vi "Test InfluxDB Client.vi"() -> ()   [LabVIEW 2015]
doc: "Test program for the InfluxDB client."
uses:
  Schema.ctl
  InfluxDB Client/InfluxDB Client.lvclass
  InfluxDB Client/Time precision.ctl
panel:
  out "Data out":T1[](array[typedef]) {"time" format="%<%I:%M:%S%3u %p\n%Y/%m/%d>T"}
  in  "Data in":T1[](array[typedef])=[{"time"=timestamp(3513058155.541 s since 1904-01-01), "string"="textA", "extended"=1.234, "double"=1.23, "single"=1.2, "int64"=-64, "int32"=-32, "int16"=-16, "int8"=-8, "uint64"=64, "uint32"=32, "uint16"=16, "uint8"=8, "boolean"=TRUE}, {"time"=timestamp(3511762155.542 s since 1904-01-01), "string"="textB", "extended"=-1.234, "double"=-1.23, "single"=-1.2, "int64"=1, "int32"=2, "int16"=3, "int8"=4, "uint64"=5, "uint32"=6, "uint16"=7, "uint8"=8, "boolean"=FALSE}] {"time" format="%<%I:%M:%S%3u %p\n%Y/%m/%d>T"}
  out "Time series names":string[](array[string])
  out "Database names":string[](array[string])
  out "Ping status":string
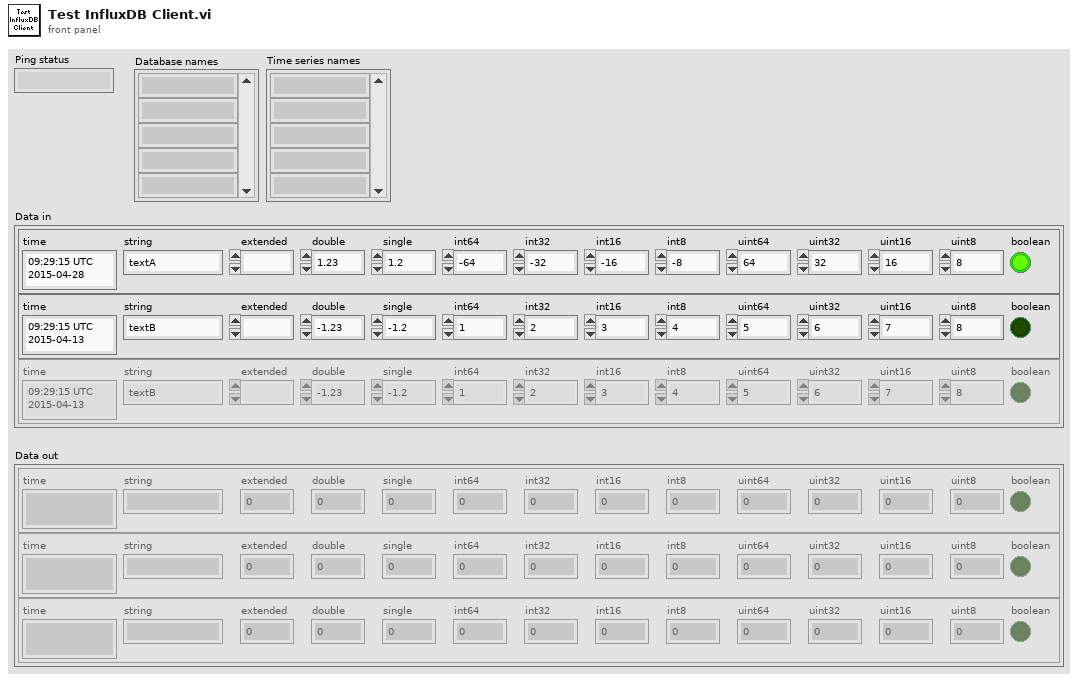
[diagram p1: front panel]
types:
  T1 = typedef "Schema.ctl" = cluster{"time":timestamp, "string":string, "extended":ext, "double":dbl, "single":sgl, "int64":i64, "int32":i32, "int16":i16, "int8":i8, "uint64":u64, "uint32":u32, "uint16":u16, "uint8":u8, "boolean":bool}
  T2 = typedef "InfluxDB Client.lvclass/Time precision.ctl" = enum16{"seconds", "milliseconds", "microseconds"}
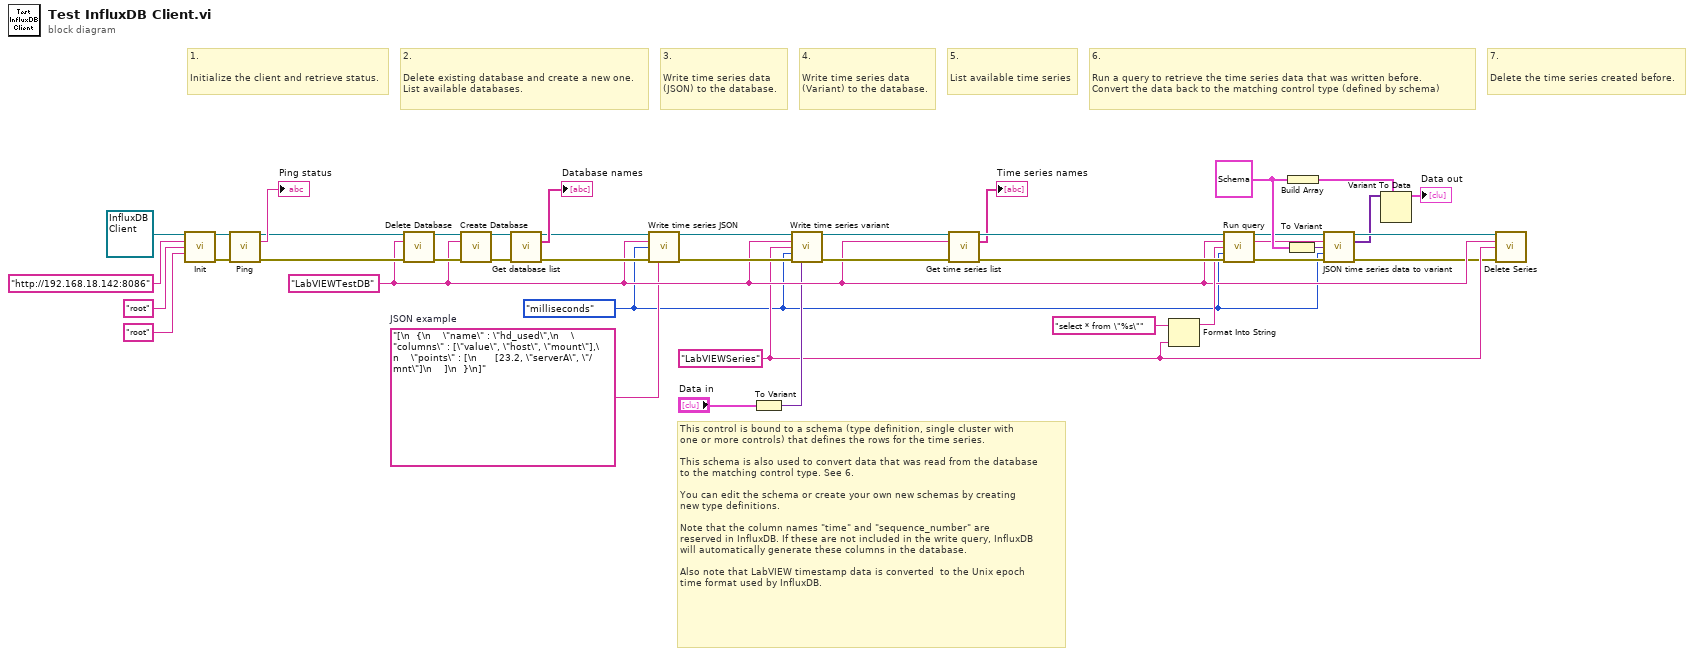
[diagram p0: block diagram]
diagram:
  w9 = "[\n  {\n    \"name\" : \"hd_used\",\n    \"columns\" : [\"value\", \"host\", \"mount\"],\n    \"points\" : [\n      [23.2, \"serverA\", \"/mnt\"]\n    ]\n  }\n]"  # JSON example
  w8 = "LabVIEWSeries" ("Url")
  w21 = T1 {"time"=timestamp(0 s since 1904-01-01), "string"="", "extended"=0.0, "double"=0.0, "single"=0.0, "int64"=0, "int32"=0, "int16"=0, "int8"=0, "uint64"=0, "uint32"=0, "uint16"=0, "uint8"=0, "boolean"=FALSE} ("Schema")
  w1 = Time_precision."milliseconds" ("Precision")
  w12 = "LabVIEWTestDB" ("Url")
  # "7.\n\nDelete the time series created before."
  # "6.\n\nRun a query to retrieve the time series data that was written before.\nConvert the data back to the matching control type (defined by schema)"
  # "5.\n\nList available time series"
  # "4.\n\nWrite time series data\n(Variant) to the database."
  # "3.\n\nWrite time series data\n(JSON) to the database."
  # "2.\n\nDelete existing database and create a new one.\nList available databases."
  # "1.\n\nInitialize the client and retrieve status."
  # "This control is bound to a schema (type definition, single cluster with\none or more controls) that defines the rows for the time series.\n\nThis schema is also used to convert data that was read from the database\nto the matching control type. See 6.\n\nYou can edit the schema or create your own new schemas by creating\nnew type definitions.\n\nNote that the column names \"time\" and \"sequence_number\" are\nreserved in InfluxDB. If these are not included in the write query, InfluxDB\nwill automatically generate these columns in the database.\n\nAlso note that LabVIEW timestamp data is converted  to the Unix epoch\ntime format used by InfluxDB."
  n1 = call "Init.vi"("InfluxDB in"=refnum<class "InfluxDB Client.lvclass"> refnum, "Url"="http://192.168.18.142:8086", "Username"="root" ("Url"), "Password"="root" ("Url")) -> ("InfluxDB out"=w39:refnum<class "InfluxDB Client.lvclass">, "error out"=w38:errorcluster)  [unwired: 10 in]
  n2 = call "Ping.vi"("InfluxDB in"=w39, "error in (no error)"=w38) -> ("InfluxDB out"=w14:refnum<class "InfluxDB Client.lvclass">, "Ping status"=→"Ping status":string, "error out"=w13:errorcluster)  [unwired: 11 in]
  n3 = call "Delete Database.vi"("InfluxDB in"=w14, "Database name"=w12, "error in (no error)"=w13) -> ("InfluxDB out"=w33:refnum<class "InfluxDB Client.lvclass">, "error out"=w32:errorcluster)  [unwired: 11 in]
  n4 = call "Create Database.vi"("InfluxDB in"=w33, "Database name"=w12, "error in (no error)"=w32) -> ("InfluxDB out"=w27:refnum<class "InfluxDB Client.lvclass">, "error out"=w28:errorcluster)  [unwired: 11 in]
  n5 = call "Get database list.vi"("InfluxDB in"=w27, "error in (no error)"=w28) -> ("InfluxDB out"=w25:refnum<class "InfluxDB Client.lvclass">, "Database names"=→"Database names":string[], "error out"=w24:errorcluster)  [unwired: 11 in]
  n6 = call "Write time series JSON.vi"("InfluxDB in"=w25, "Database name"=w12, "Precision (ms)"=w1, "error in (no error)"=w24, "JSON data"=w9) -> ("InfluxDB out"=w18:refnum<class "InfluxDB Client.lvclass">, "error out"=w16:errorcluster)  [unwired: 9 in]
  n7 = To Variant(anything="Data in") -> (Variant=w11:variant)
  n8 = call "Write time series variant.vi"("InfluxDB in"=w18, "Database name"=w12, "Series name"=w8, "Precision (ms)"=w1, "error in (no error)"=w16, "Variant data"=w11) -> ("InfluxDB out"=w17:refnum<class "InfluxDB Client.lvclass">, "error out"=w15:errorcluster)  [unwired: 8 in]
  n9 = call "Get time series list.vi"("InfluxDB in"=w17, "Database name"=w12, "error in (no error)"=w15) -> ("InfluxDB out"=w30:refnum<class "InfluxDB Client.lvclass">, "Time series names"=→"Time series names":string[], "error out"=w31:errorcluster)  [unwired: 10 in]
  n10 = Format Into String(format string="select * from \"%s\"" ("Url"), w8) -> (resulting string=w22:string)  [unwired: 2 in, 1 out]
  n11 = call "Run query.vi"("InfluxDB in"=w30, "Database name"=w12, "Query"=w22, "Precision (ms)"=w1, "error in (no error)"=w31) -> ("InfluxDB out"=w7:refnum<class "InfluxDB Client.lvclass">, "JSON data"=w6:string, "error out"=w3:errorcluster)  [unwired: 8 in]
  n12 = To Variant(anything=w21) -> (Variant=w5:variant)
  n13 = Build Array(w21) -> (w20:T1[])
  n14 = call "JSON time series data to variant.vi"("InfluxDB in"=w7, "JSON data"=w6, "Schema"=w5, "Precision (ms)"=w1, "error in (no error)"=w3) -> ("Data (variant)"=w4:variant[], "error out"=w2:errorcluster)  [unwired: 8 in, 1 out]
  n15 = Variant To Data(type=w20, Variant=w4) -> (data=→"Data out":T1[])  [unwired: 1 in, 1 out]
  n16 = call "Delete Series.vi"("InfluxDB in"=w7, "Database name"=w12, "Series name"=w8, "error in (no error)"=w2) -> ()  [unwired: 10 in, 2 out]
